vi "libssh2_channel_close.vi"(8 "error in (no error)":errorcluster, 11 "channel":T1) -> (0 "error out":errorcluster)   [LabVIEW 2013, in "libssh2.lvlib"]
doc: "Closes an active data channel. In practice this means sending an SSH_MSG_CLOSE packet to the remote host which serves as instruction that no further data will be sent to it. The remote host may still send data back until it sends its own message in response. To wait for the remote end to close its connection as well, follow this command with 'libssh2_channel_wait_closed'."
uses:
  libssh2.lvlib
  Channel Refnum.ctl
  Not A Channel.vi
  <vilib>/Utility/error.llb/Error Cluster From Error Code.vi
  Global Settings.vi
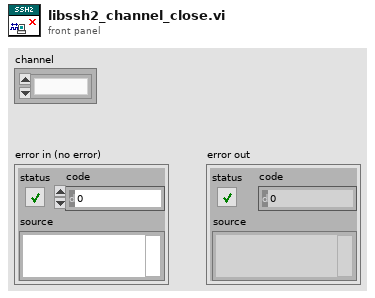
[diagram p1: front panel]
types:
  T1 = typedef "libssh2.lvlib/Channel Refnum.ctl" = refnum<k1>
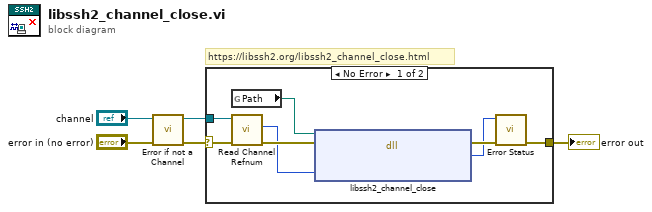
[diagram p0: block diagram]
diagram:
  # "https://libssh2.org/libssh2_channel_close.html"
  n1 = call "Error if not a Channel.vi"("error in (no error)"="error in (no error)", "channel"="channel") -> ("error out"=w3:errorcluster, "channel out"=w1:T1)  [unwired: 8 in]
  n2 = case shown="No Error" w3 {
    selector: w3 -> [w13 w14]
    tunnel: [w12 w14] -> w5
    tunnel: w1 -> [w11 _]
    frame No Error {
      n3 = global read "Global Settings.vi" "Path"() -> (w7:path)
      n4 = call "Read Channel Refnum.vi"("error in (no error)"=w13, "channel"=w11) -> ("error out"=w9:errorcluster, "LIBSSH2_CHANNEL*"=w8:u64)  [unwired: 8 in]
      n5 = dll-call lib="?" fn="libssh2_channel_close"(path in=w7, error in=w9, "channel"=w8) -> (error out=w10:errorcluster, "return value"=w6:i32)  [unwired: 2 in, 1 out]
      n6 = call "Error Status.vi"("error in (no error)"=w10, "return value"=w6) -> ("error out"=w12:errorcluster)  [unwired: 8 in, 1 out]
    }
    frame Error {
    }
  }
  "error out" <- w5
